vi "ABR-Initialize.vi"(0 "Params":T3={"CAP or ABR"=enum."ABR", "Stimulus"={"Ear"=enum."Left", "Start (dB)"=0, "Waveform"=enum."TONE PIP", "Stop (dB)"=30, "Frequency (kHz)"=16.0, "Step (dB)"=5, "Rep rate (/sec)"=30.0, "Alternate Polarity"=FALSE}, "Response"={"Gain"=10000, "Averages"=512, "Window (ms)"=8.5, "Thr Fast Steps"=8.5}, "Hidden"={"AI Samp Rate Hz"=25000.0, "AO Samp Rate Hz"=100000.0, "Duration (ms)"=5.0, "Ramp (ms)"=0.5, "Click width (us)"=0.0, "ITI"=enum."Rate", "Save raw"=FALSE}, "Version"=0} {"Response"."Thr Fast Steps" format="%.2f"; "Response"."Window (ms)" format="%.2f"; "Stimulus"."Frequency (kHz)" format="%.2f"; "Stimulus"."Start (dB)" step=5}, 1 "State":T8) -> (4 "Runtime":T7, 13 "Analysis":T1, 14 "Ceiling":dbl, 15 "error out":errorcluster)   [LabVIEW 2020]
uses:
  Threshold Estimation VIs/ABR3-Threshold Estimation Result.ctl
  Typedefs/ABR-Response.ctl
  Typedefs/ABR-Stimulus.ctl
  CFTS SubVIs/CFTS-Experiment State.ctl
  Typedefs/ABR-Hidden Params.ctl
  Typedefs/ABR-Runtime Data.ctl
  Typedefs/ABR-Parameters.ctl
  Typedefs/ABR-Analysis State.ctl
panel:
  in  "error in (no error)":errorcluster
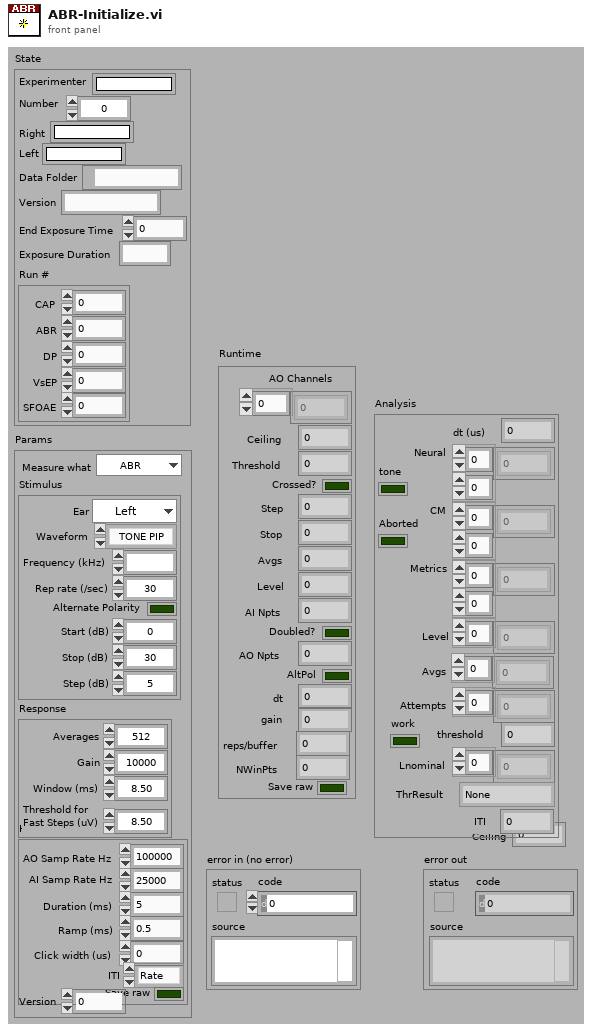
[diagram p1: front panel]
types:
  T1 = typedef "ABR-Analysis State.ctl" = cluster{"dt (us)":dbl, "Neural":dbl[][], "CM":dbl[][], "Metrics":dbl[][], "Level":dbl[], "Avgs":i32[], "Attempts":i32[], "Aborted":bool, "threshold":dbl, "Lnominal":dbl[], "tone":bool, "work":bool, "ThrResult":T2, "ITI":dbl}
  T2 = typedef "ABR3-Threshold Estimation Result.ctl" = enum16{"None", "Power", "Sigmoid", "Power (noisy)", "Suprathreshold", "Invalid"}
  T3 = typedef "ABR-Parameters.ctl" = cluster{"CAP or ABR":enum16{"CAP", "ABR"}, "Stimulus":T4, "Response":T5, "Hidden":T6, "Version":i32}
  T4 = typedef "ABR-Stimulus.ctl" = cluster{"Ear":enum16{"Right", "Left", "Bone"}, "Start (dB)":i32, "Waveform":enum16{"TONE PIP", "CLICK"}, "Stop (dB)":i32, "Frequency (kHz)":ext, "Step (dB)":i32, "Rep rate (/sec)":dbl, "Alternate Polarity":bool}
  T5 = typedef "ABR-Response.ctl" = cluster{"Gain":i32, "Averages":i32, "Window (ms)":sgl, "Thr Fast Steps":sgl}
  T6 = typedef "ABR-Hidden Params.ctl" = cluster{"AI Samp Rate Hz":dbl, "AO Samp Rate Hz":dbl, "Duration (ms)":dbl, "Ramp (ms)":dbl, "Click width (us)":dbl, "ITI":enum16{"Rate", "Interval"}, "Save raw":bool}
  T7 = typedef "ABR-Runtime Data.ctl" = cluster{"AO Channels":i32[], "Ceiling":dbl, "Threshold":dbl, "Crossed?":bool, "Step":dbl, "Stop":i32, "Avgs":i32, "Level":dbl, "AI Npts":i32, "Doubled?":bool, "AO Npts":i32, "AltPol":bool, "dt":dbl, "gain":dbl, "reps/buffer":i32, "NWinPts":i32, "Save raw":bool}
  T8 = typedef "CFTS-Experiment State.ctl" = cluster{"Experimenter":string, "Number":u32, "Right":string, "Left":string, "Data Folder":path, "Version":string, "End Exposure Time":dbl, "Exposure Duration":string, "Run #":cluster{"CAP":i32, "ABR":i32, "DP":i32, "VsEP":i32, "SFOAE":i32}}
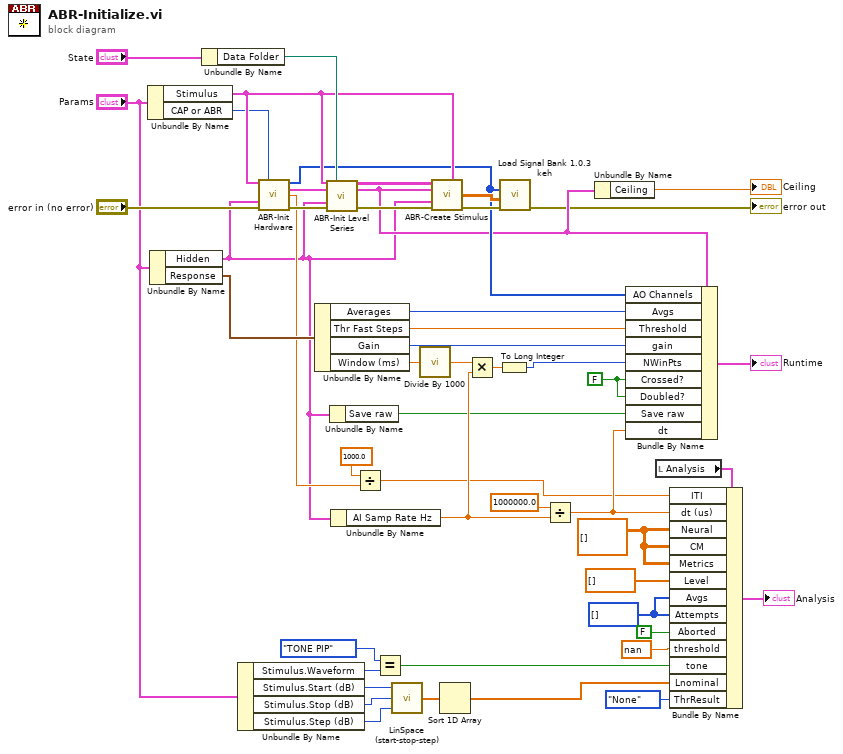
[diagram p0: block diagram]
diagram:
  w29 = i32[] [] ("Avgs")
  w31 = dbl[][] [] ("Neural")
  w37 = FALSE ("Crossed?")
  n1 = Unbundle By Name("Params") -> ("Stimulus"=w36:T4, "CAP or ABR"=w35:enum16{"CAP", "ABR"})
  n2 = Unbundle By Name("Params") -> ("Hidden"=w2:T6, "Response"=w34:T5)
  n3 = Unbundle By Name("State") -> ("Data Folder"=w45:path)
  n4 = Unbundle By Name("Params") -> ("Stimulus.Waveform"=w16:enum16{"TONE PIP", "CLICK"}, "Stimulus.Start (dB)"=w13:i32, "Stimulus.Stop (dB)"=w12:i32, "Stimulus.Step (dB)"=w11:i32)
  n5 = call "ABR-Init Hardware.vi"("Stimulus"=w36, "CAP or ABR"=w35, "Hidden"=w2, "error in (no error)"="error in (no error)") -> ("AO Channels"=w26:i32[], "Runtime"=w25:T7, "Coerced rep rate"=w5:dbl, "error out"=w43:errorcluster)  [unwired: 8 in]
  n6 = Unbundle By Name(w34) -> ("Averages"=w40:i32, "Thr Fast Steps"=w39:sgl, "Gain"=w23:i32, "Window (ms)"=w21:sgl)
  n7 = call "ABR-Init Level Series.vi"("Stimulus"=w36, "Data Folder"=w45, "Runtime In"=w25, "Hidden"=w2) -> ("Runtime Out"=w9:T7)  [unwired: 10 in, 1 out]
  n8 = Unbundle By Name(w2) -> ("Save raw"=w1:bool)
  n9 = Unbundle By Name(w2) -> ("AI Samp Rate Hz"=w20:dbl)
  n10 = Divide(x=1000.0, y=w5) -> (x/y=w4:dbl)
  n11 = Equal?(x=enum16{"TONE PIP", "CLICK"}."TONE PIP", y=w16) -> (x = y?=w14:bool)
  n12 = call "LinSpace (start-stop-step).vi"("Step"=w11, "Stop"=w12, "Start"=w13) -> ("Array"=w10:dbl[])  [unwired: 1 in, 1 out]
  n13 = call "Divide By 1000.vi"("X"=w21) -> ("X/1000"=w19:dbl)
  n14 = call "ABR-Create Stimulus.vi"("Stimulus"=w36, "Runtime"=w9, "Hidden"=w2, "error in (no error)"=w43) -> ("stimulus"=w47:dbl[][], "error out"=w48:errorcluster)  [unwired: 10 in]
  n15 = Sort 1D Array(array=w10) -> (sorted array=w7:dbl[])
  n16 = Multiply(x=w19, y=w20) -> (x*y=w22:dbl)
  n17 = To Long Integer(number=w22) -> (32bit integer=w18:i32)
  n18 = call "Load Signal Bank 1.0.3 keh.vi"("error in (no error)"=w48, "Input array"=w47, "Active AO Array"=w26) -> ("error out"=→"error out":errorcluster)  [unwired: 6 in, 2 out]
  n19 = Divide(x=1000000.0, y=w20) -> (x/y=w24:dbl)
  n20 = Unbundle By Name(w9) -> ("Ceiling"=→"Ceiling":dbl)
  n21 = Bundle By Name(cluster=w9, "AO Channels"=w26, "Avgs"=w40, "Threshold"=w39, "gain"=w23, "NWinPts"=w18, "Crossed?"=w37, "Doubled?"=w37, "Save raw"=w1, "dt"=w24) -> (→"Runtime":T7)
  n22 = local read "Analysis"() -> (w33:T1)
  n23 = Bundle By Name(cluster=w33, "ITI"=w4, "dt (us)"=w24, "Neural"=w31, "CM"=w31, "Metrics"=w31, "Level"=dbl[] [], "Avgs"=w29, "Attempts"=w29, "Aborted"=FALSE, "threshold"=nan, "tone"=w14, "Lnominal"=w7, "ThrResult"=ABR3-Threshold_Estimation_Result."None") -> (→"Analysis":T1)
